vi "Subset Transfer Groups.vi"(8 "error in (no error)":errorcluster, 9 "count":i32, 10 "index":i32, 11 "Transfer Groups":refnum<class "Transfer Group.lvclass">[](array[class])) -> (0 "error out":errorcluster, 2 "index + count":i32, 3 "subset Transfer Groups":refnum<class "Transfer Group.lvclass">[](array[class]))   [LabVIEW 2019, in "DSF Core.lvlib" / "Transfer Group.lvclass"]
uses:
  Transfer Group.lvclass
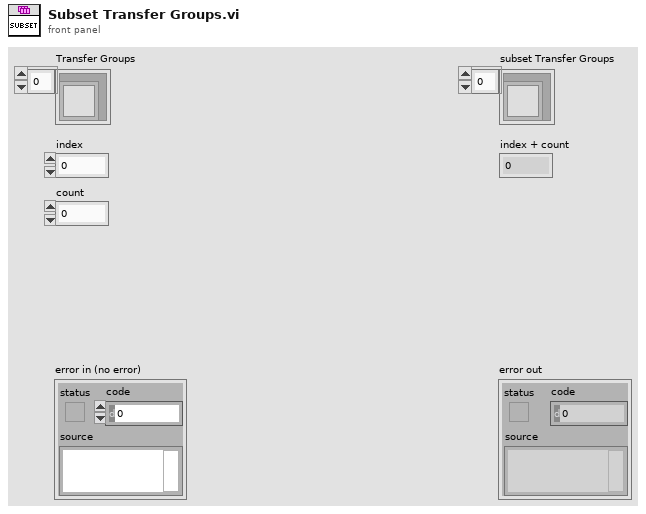
[diagram p1: front panel]
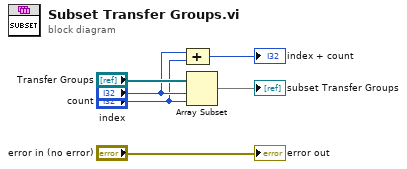
[diagram p0: block diagram]
diagram:
  n1 = Compound Arithmetic op=ADD("index", "count") -> (→"index + count":i32)
  n2 = Array Subset(array="Transfer Groups", index="index", length="count") -> (→"subset Transfer Groups":refnum<class "Transfer Group.lvclass">[])
  "error out" <- "error in (no error)"
